vi "FilteringTest.vi"() -> ()   [LabVIEW 2011]
uses:
  <vilib>/rvi/eio/common/nirviEmuTemplateMethod_errors.vi
  <vilib>/rvi/interface/RandomDataEmulation/nirviRandomDataFPGAFIFO.vi
  <vilib>/rvi/interface/RandomDataEmulation/niFpgaRandomDataHandleErrors.vi
  <vilib>/eio/EIONode/EIONode.xnode
  <vilib>/rvi/Analysis/measure/butterworth/XNode/niFpgaButterworthFilter.xnode
  <vilib>/rvi/DataTransferAndStorage/Container/XNode/niFpgaContainer.xnode
  <vilib>/rvi/interface/RandomDataEmulation/nirviRandomDataFpgaReadWriteTemplate.vi
panel:
  out "integer 2":i32
  in  "Filter":bool
  out "Timed Out?":bool
  out "LoopTickTime":u32
  in  "stop":bool
  out "integer":i64
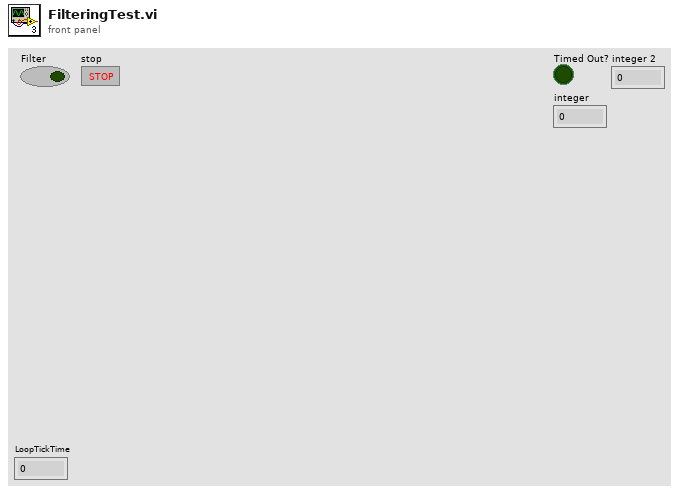
[diagram p1: front panel]
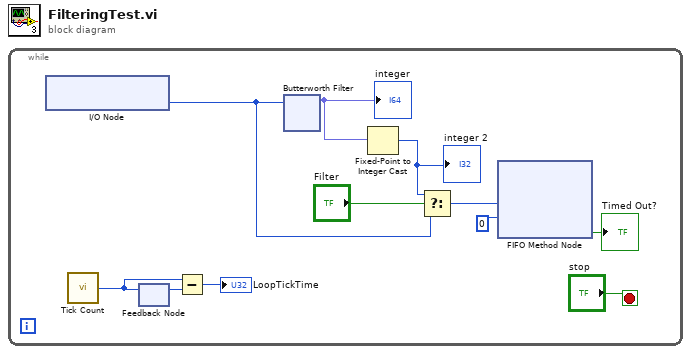
[diagram p0: block diagram]
diagram:
  n1 = while {
    stop <- "stop" stop-if-true
    n2 = xnode "I/O Node"() -> ("IO Module\\AI A0"=w2:i16)  [unwired: 1 in, 1 out]
    n3 = call "Tick Count"() -> ("Tick Count(Ticks)"=w9:u32)
    n4 = feedback #1() -> (w8:u32)  [unwired: 1 in]
    n5 = feedback-in #1(w9) -> ()
    n6 = Subtract(x=w9, y=w8) -> (x-y=→"LoopTickTime":u32)
    n7 = xnode "Butterworth Filter"("input data"=w2) -> ("output data"=w5:fxp<+/-,20,20>)  [unwired: 2 in]
    "integer" <- w5
    n8 = Fixed-Point to Integer Cast(1:w5) -> (0:w4:i32)
    "integer 2" <- w4
    n9 = Select(t=w4, s="Filter", f=w2) -> (s? t:f=w3:i32)
    n10 = xnode ("FIFO Method Node")("Element"=w3, "Timeout"=0) -> ("Timed Out?"=→"Timed Out?":bool)  [unwired: 1 in, 1 out]
  }
